vi "test_PlaceLeftOfvalidation.vi"(11 "Test Case In":refnum<class "RelativePlacingTests.lvclass">) -> (0 "error out":errorcluster, 3 "Test Case Out":refnum<class "RelativePlacingTests.lvclass">)   [LabVIEW 2023, in "RelativePlacingTests.lvclass"]
uses:
  RelativePlacingTests.lvclass
  <vilib>/Astemes/LUnit/Test Case.lvclass/Test Case.ctl
  <vilib>/Astemes/LUnit/Core/LUnit Test Case/Private/Append Fail Result.vi
  <vilib>/Astemes/LUnit/Core/LUnit Test Case/Private/Append Pass Result.vi
  <vilib>/Astemes/LUnit/Core/LUnit Test Case/Private/Run In UI.vi
  <vilib>/Utility/error.llb/Clear Errors.vi
  RelativePlacingTests.lvclass/RelativePlacingTests.ctl
  <vilib>/Astemes/LUnit/Test Case.lvclass
panel:
  in  "movingObject":string
  in  "anchor":dbl
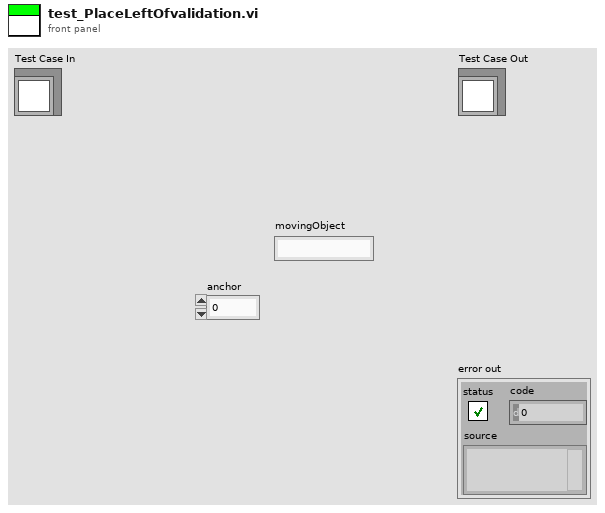
[diagram p1: front panel]
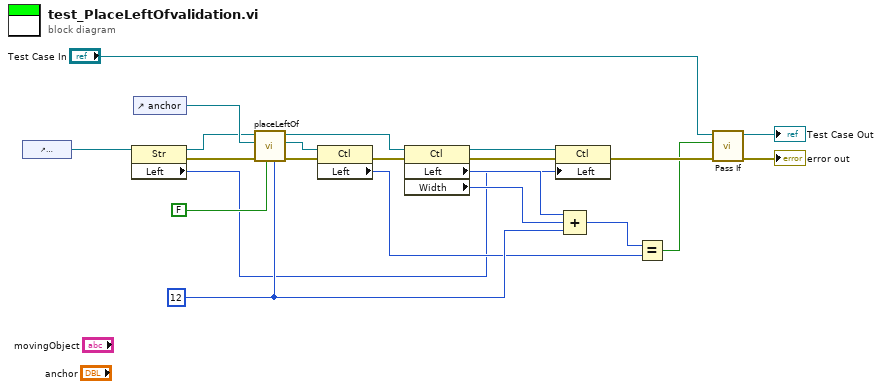
[diagram p0: block diagram]
diagram:
  w14 = u16 12 ("spacing")
  n1 = control-ref of="movingObject"() -> (w7:refnum<vi>)
  n2 = property class="Str"(reference=w7) -> (reference out=w6:refnum<vi>, error out=w17:errorcluster, "Left"=w2:i32)  [unwired: 1 in]
  n3 = control-ref of="anchor"() -> (w18:refnum<vi>)
  n4 = call "placeLeftOf.vi"("spacing"=w14, "useControlBodyOnly"=FALSE, "error in (no error)"=w17, "anchorObject"=w18, "movingObject"=w6) -> ("error out"=w13:errorcluster, "anchorObject(dup)"=w11:refnum<vi>, "movingObject(dup)"=w10:refnum<vi>)  [unwired: 4 in]
  n5 = property class="Ctl"(reference=w11, error in=w13) -> (error out=w12:errorcluster, "Left"=w4:i32)  [unwired: 1 out]
  n6 = property class="Ctl"(reference=w10, error in=w12) -> (reference out=w8:refnum<vi>, error out=w9:errorcluster, "Left"=w16:i32, "Width"=w15:u32)
  n7 = property class="Ctl"(reference=w8, error in=w9, "Left"=w2) -> (error out=w3:errorcluster)  [unwired: 1 out]
  n8 = Compound Arithmetic op=ADD(w16, w15, w14) -> (w5:u32)
  n9 = Equal?(x=w5, y=w4) -> (x = y?=w1:bool)
  n10 = call <vilib>:"Pass If.vi"("error in (no error)"=w3, "Pass?"=w1, "LUnit Test Case In"="Test Case In") -> ("error out"=→"error out":errorcluster, "LUnit Test Case Out"=→"Test Case Out":refnum<class "RelativePlacingTests.lvclass">)  [unwired: 7 in]
